vi "BrightnessSettings.vi"(10 "error in (no error)":errorcluster, 11 "Refnum in":T2) -> (2 "error out":errorcluster, 3 "Refnum out":T2)   [LabVIEW 2014]
uses:
  <vilib>/userdefined/High Color/VBAIInterface.ctl
  c_VBAI_SelcectInspection.ctl
  g_Stop.vi
panel:
  in  "OK":bool
  out "Template":picture
  out "Camera Image":T1(plugin-control)
  out "Inspection Status":bool
  # "Adjust the brightness of the light source and the camera focus until the Camera Image looks similar to the Template. The LED indicates if the adjustment process would pass or not.\n(The chip might have to be moved in order to recognize the pattern and display the PASS status)"
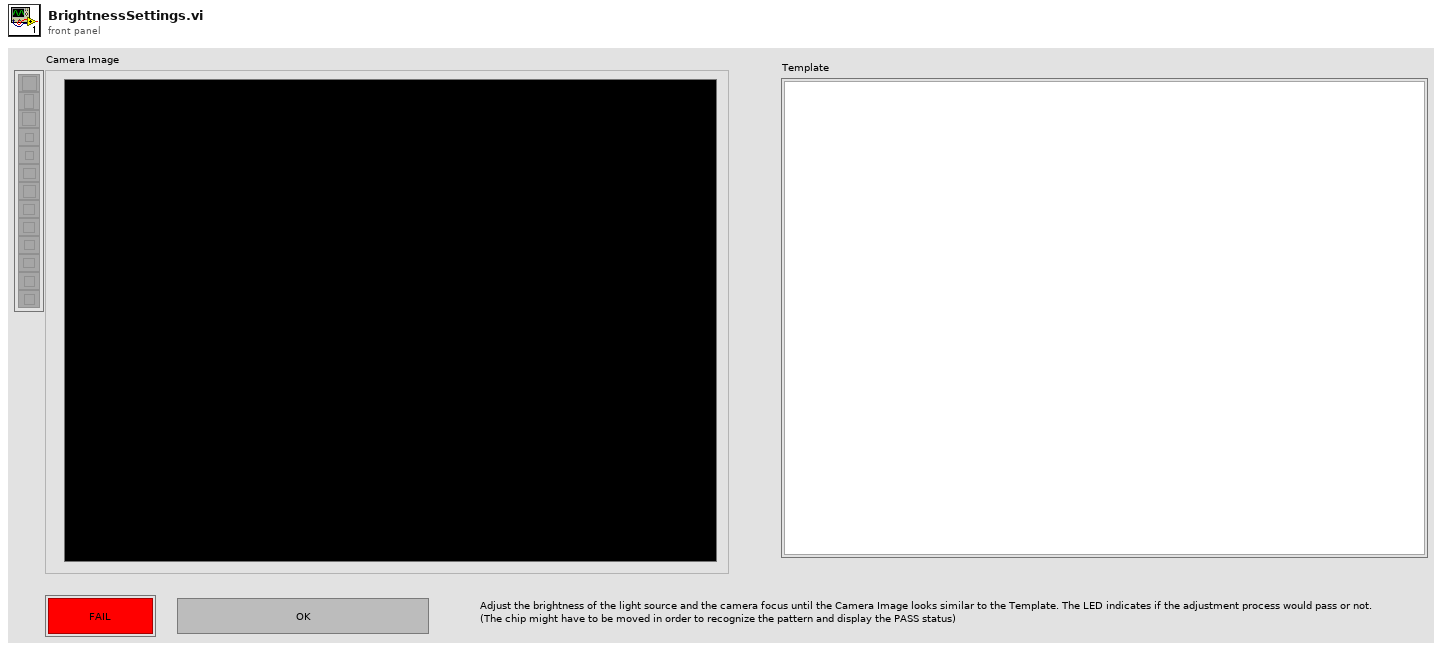
[diagram p1: front panel]
types:
  T1 = typedef "IMAQ Image.ctl" = refnum<image>
  T2 = typedef "VBAIInterface.ctl" = refnum<k21>
  T3 = typedef "c_VBAI_SelcectInspection.ctl" = enum16{"Image Acquisition", "Find Reference", "Chip Alignment", "Adjustment", "Porbecard Positioning"}
  T4 = cluster{"PASS/FAIL Flag":bool, "Numeric Measurement":dbl, "String Measurement":string, "Report Text":string}
  T5 = enum32{"invalid app kind", "Development System", "Run Time System", "Student Edition", "Embedded LabVIEW", "Evaluation", "Custom"}
  T6 = typedef "imagedata.ctl" = cluster{"image type":i32, "image depth":i32, "image":u8[], "mask":u8[], "colors":u32[], "Rectangle":cluster{"left":i16, "top":i16, "right":i16, "bottom":i16}}
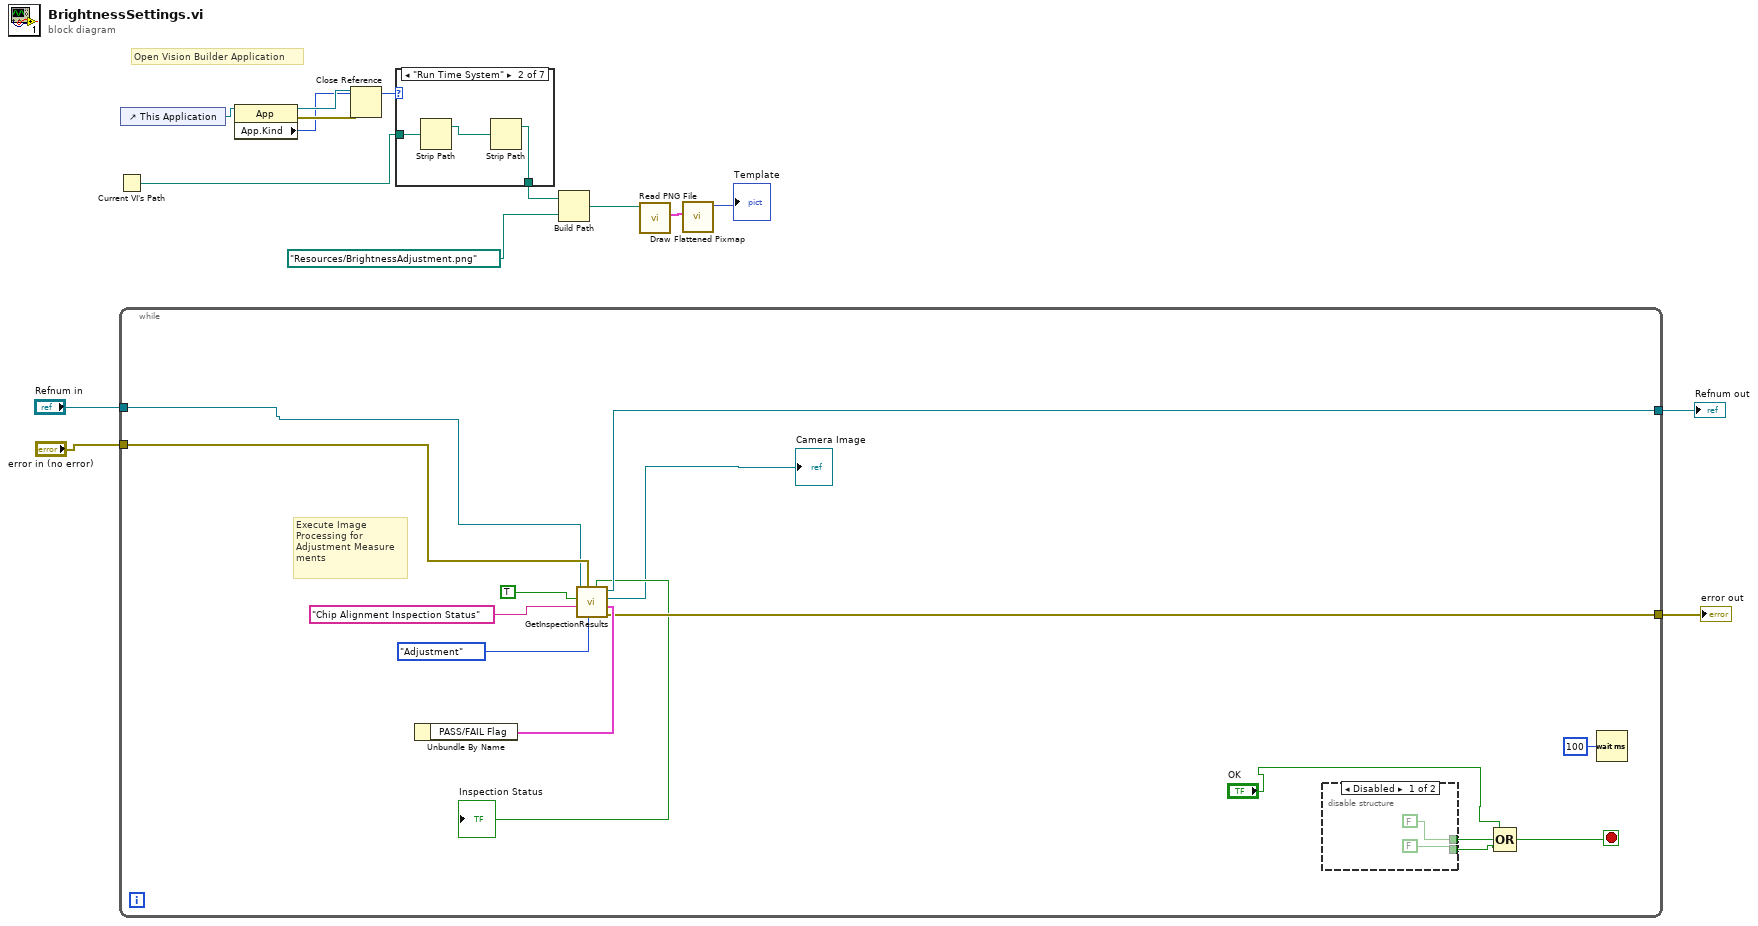
[diagram p0: block diagram]
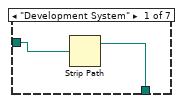
[diagram p2: hidden frame]
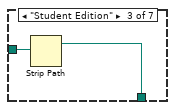
[diagram p3: hidden frame]
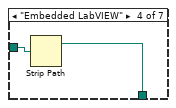
[diagram p4: hidden frame]
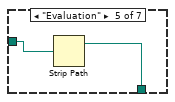
[diagram p5: hidden frame]
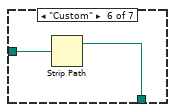
[diagram p6: hidden frame]
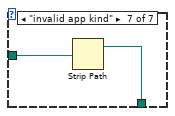
[diagram p7: hidden frame]
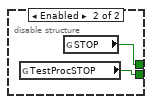
[diagram p8: hidden frame]
diagram:
  # "Open Vision Builder Application"
  n1 = Current VI's Path() -> (path=w6:path)
  n2 = while {
    tunnel: "error in (no error)" -> [w24]
    tunnel: "Refnum in" -> [w23]
    tunnel: [w22] -> w12
    tunnel: [w21] -> w11
    stop <- w16 stop-if-true
    # "Execute Image\nProcessing for\nAdjustment Measure\nments"
    n3 = call "GetInspectionResults.vi"("Select Inspection"=c_VBAI_SelcectInspection."Adjustment", "error in (no error)"=w24, "StepName"="Chip Alignment Inspection Status", "Image Enable"=TRUE, "Refnum in"=w23) -> ("error out"=w21:errorcluster, "Results"=w26:T4, "Image Dst Out"=→"Camera Image":T1, "Refnum out"=w22:T2, "Inspection Status"=→"Inspection Status":bool)  [unwired: 2 in]
    n4 = Unbundle By Name(w26) -> ()  [unwired: 1 out]
    n5 = disable-structure shown="Disabled" {
      disable-tunnel: [FALSE w33] -> w18
      disable-tunnel: [FALSE w32] -> w17
      frame Disabled {
      }
      frame Enabled {
        n6 = global read "g_Stop.vi" "TestProcSTOP"() -> (w32:bool)
        n7 = global read "g_Stop.vi" "STOP"() -> (w33:bool)
      }
    }
    n8 = Compound Arithmetic op=OR("OK", w18, w17) -> (w16:bool)
    n9 = Wait (ms)(milliseconds to wait=u32 100) -> ()  [unwired: 1 out]
  }
  "Refnum out" <- w12
  "error out" <- w11
  n10 = control-ref of="This Application"() -> (w8:refnum<vi>)
  n11 = property class="App"(reference=w8) -> (reference out=w10:refnum<vi>, error out=w9:errorcluster, "App.Kind"=w7:T5)  [unwired: 1 in]
  n12 = Close Reference(reference=w10, error in (no error)=w9) -> ()  [unwired: 1 out]
  n13 = case shown="\"Run Time System\"" w7 {
    tunnel: w6 -> [w35 w38 w40 w42 w44 w46 w47]
    tunnel: [w34 w36 w39 w41 w43 w45 w48] -> w5
    frame "Development System" {
      n14 = Strip Path(path=w35) -> (stripped path=w34:path)  [unwired: 1 out]
    }
    frame "Run Time System" {
      n15 = Strip Path(path=w38) -> (stripped path=w37:path)  [unwired: 1 out]
      n16 = Strip Path(path=w37) -> (stripped path=w36:path)  [unwired: 1 out]
    }
    frame "Student Edition" {
      n17 = Strip Path(path=w40) -> (stripped path=w39:path)  [unwired: 1 out]
    }
    frame "Embedded LabVIEW" {
      n18 = Strip Path(path=w42) -> (stripped path=w41:path)  [unwired: 1 out]
    }
    frame "Evaluation" {
      n19 = Strip Path(path=w44) -> (stripped path=w43:path)  [unwired: 1 out]
    }
    frame "Custom" {
      n20 = Strip Path(path=w46) -> (stripped path=w45:path)  [unwired: 1 out]
    }
    frame "invalid app kind" {
      n21 = Strip Path(path=w47) -> (stripped path=w48:path)  [unwired: 1 out]
    }
  }
  n22 = Build Path(base path=w5, name or relative path=path "Resources/BrightnessAdjustment.png") -> (appended path=w1:path)
  n23 = call <vilib>:"Read PNG File.vi"("path to PNG file"=w1) -> ("image data"=w4:T6)  [unwired: 8 in, 2 out]
  n24 = call <vilib>:"Draw Flattened Pixmap.vi"("image data"=w4) -> ("new picture"=→"Template":picture)  [unwired: 8 in]
